vi "CRYRead COM Port.vi"(6 "Current seq step setups":string[](array[string]), 7 "Serial Port":u8=2 max=4, 8 "Hardware setup (if array not wired)":string, 10 "Status Line 2":enum16{"CTS", "DSR", "RI", "CD"}(ring), 11 "Status Line":enum16{"CTS", "DSR", "RI", "CD"}(ring)=enum."DSR") -> (2 "State 2 (Start & Continue)":bool, 3 "State (Redo & Abort)":bool, 5 "Registers":bool[](array[boolean])=[FALSE, FALSE, FALSE, FALSE, FALSE, FALSE, FALSE, FALSE, FALSE, TRUE, TRUE, FALSE, FALSE, FALSE, FALSE, FALSE])   [LabVIEW 2013]
doc: "This VI returns the state of the specified status lines of a serial port."
uses:
  Task Sequence/CRYProject Run Control Global.vi
panel:
  # "Note:  This new version uses VISA calls and requires VISA drivers to be installed."
  # "Modem Status Registers"
  # "15"
  # "0"
  # "Status Registers\n(base adr + 5)"
  # "CTS - Connect the footswitch across pins 8&7 (white & grey)"
  # "DSR - Connect the footswitch across pins 6&7 (blue & grey)"
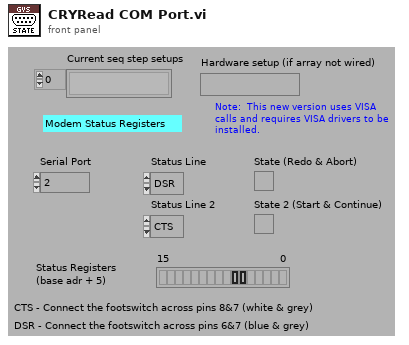
[diagram p1: front panel]
types:
  T1 = typedef "CRYHardware.ctl" = cluster{"Name":string, "Analog I/O":u16, "Digital I/O":u16, "Channels":u8, "Dig Dev ID":u8, "N ports":u8, "Interface":u32, "Dig I/O Ports":cluster{"port #":i16, "width":i16, "direction":i32}[], "Interf settings":cluster{"Type":u16, "COM Port":u8, "Baud rate":u32, "Data bits":u32, "Parity":u16, "Stop bits":u16, "Flow control":u16, "Dev ID IEEE":u8}[], "N interfs":i32, "udev SNs":i16[], "udev enable":bool, "Channel Array":T2[], "Cal sequence":string, "SelectedIn":u16, "SelectedOut":u16, "SelectedTab":u16, "State":bool, "Help":string, "Advanced":bool, "In Audio Driver":u16, "Out Audio Driver":u16}
  T2 = typedef "CRYHardware Channel Info.ctl" = cluster{"ID":i32, "Name":string, "Digital":bool, "Input":bool, "Device Name":string, "Hardware Ch ID":u8, "Vmax (V)":dbl, "Latency (samples)":dbl, "Sampling Rate (Hz)":u32, "Bit Depth":u32, "Anti-aliasing Factor (%fs)":sgl, "DAQmx Channel":tag, "term config":i32, "Coupling":i32, "IEPE en":bool, "ASIOChannel Name":string, "Audio Driver":u16, "ASIOChannel Index":u8}
  T3 = cluster{"Type":u16, "COM Port":u8, "Baud rate":u32, "Data bits":u32, "Parity":u16, "Stop bits":u16, "Flow control":u16, "Dev ID IEEE":u8}[]
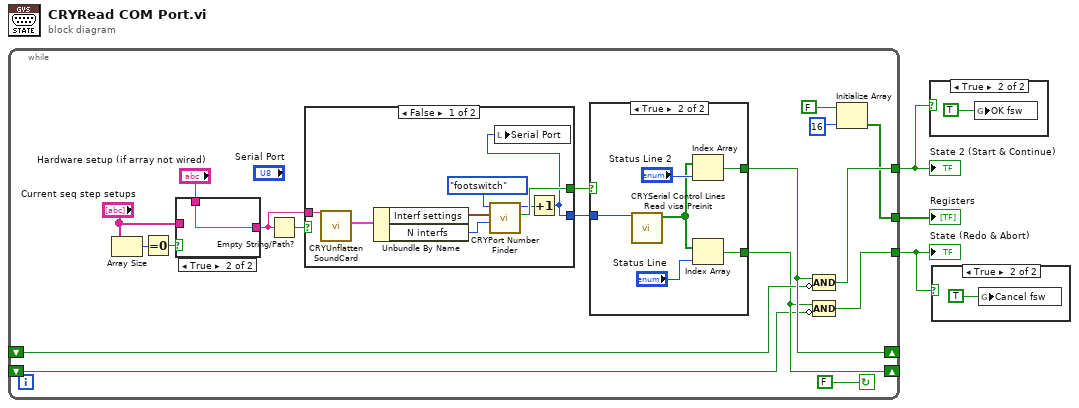
[diagram p0: block diagram]
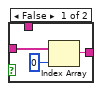
[diagram p2: hidden frame]
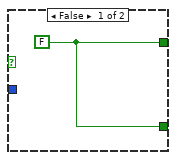
[diagram p3: hidden frame]
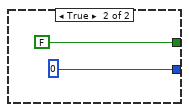
[diagram p4: hidden frame]
diagram:
  n1 = while {
    shift-left: _ -> [w10]
    shift-right: [w11] -> _
    shift-left: _ -> [w12]
    shift-right: [w13] -> _
    tunnel: [w8] -> w2
    tunnel: [w5] -> w3
    tunnel: [w9] -> w1
    stop <- FALSE continue-if-true
    n2 = Array Size(array="Current seq step setups") -> (size(s)=w16:i32)
    n3 = Equal To 0?(x=w16) -> (x = 0?=w15:bool)
    n4 = case shown="True" w15 {
      tunnel: [w23 w25] -> w21
      tunnel: "Current seq step setups" -> [w22 _]
      tunnel: "Hardware setup (if array not wired)" -> [_ w25]
      frame False {
        n5 = Index Array(array=w22, index=0) -> (element=w23:string)
      }
      frame True {
      }
    }
    n6 = Empty String/Path?(string/path=w21) -> (empty?=w19:bool)
    n7 = case shown="False" w19 {
      tunnel: [w34 u8 0] -> w20
      tunnel: w21 -> [w40 _]
      tunnel: [w36 FALSE] -> w18
      frame False {
        n8 = call "CRYUnflatten SoundCard.vi"("Flatten SoundCard"=w40) -> ("SoundCard"=w33:T1)  [unwired: 10 out]
        n9 = Unbundle By Name(w33) -> ("Interf settings"=w39:T3, "N interfs"=w38:i32)
        n10 = call "CRYPort Number Finder.vi"("N interfs"=w38, "Interf settings"=w39, "RS-232 type"=enum16{"comm", "footswitch", "buzzer"}."footswitch") -> ("Such a port exists"=w36:bool, "Port (LV)"=w35:i32)  [unwired: 7 out]
        n11 = Increment(x=w35) -> (x+1=w34:i32)
        n12 = local write "Serial Port"(w34) -> ()
      }
      frame True {
      }
    }
    n13 = case shown="True" w18 {
      tunnel: w20 -> [_ w32]
      tunnel: [w26 w28] -> w13
      tunnel: [w26 w27] -> w11
      frame False {
        w26 = FALSE
      }
      frame True {
        n14 = call "CRYSerial Control Lines Read visa Preinit.vi"("COM port (1 = COM1, etc.)"=w32) -> ("Line states (CTS, DSR, RI, DCD)"=w29:bool[])  [unwired: 10 out]
        n15 = Index Array(array=w29, index="Status Line 2") -> (element=w28:bool)
        n16 = Index Array(array=w29, index="Status Line") -> (element=w27:bool)
      }
    }
    n17 = Compound Arithmetic op=AND(w13, invert w12) -> (w9:bool)
    n18 = Compound Arithmetic op=AND(w11, invert w10) -> (w8:bool)
    n19 = Initialize Array(FALSE, 16) -> (w5:bool[])
  }
  "State 2 (Start & Continue)" <- w1
  "State (Redo & Abort)" <- w2
  "Registers" <- w3
  n20 = case shown="True" w1 {
    frame False {
    }
    frame True {
      n21 = global write "CRYProject Run Control Global.vi" "OK fsw"(TRUE ("OK fsw")) -> ()
    }
  }
  n22 = case shown="True" w2 {
    frame False {
    }
    frame True {
      n23 = global write "CRYProject Run Control Global.vi" "Cancel fsw"(TRUE ("Cancel fsw")) -> ()
    }
  }
